vi "Exercise2.3-Data Acquisition - AM.vi"() -> ()   [LabVIEW 2013]
uses:
  <vilib>/Analysis/4window.llb/windowTd.ctl
  <vilib>/measure/maspectr.llb/FFT Power Spectrum and PSD for 1 Chan (CDB).vi
  <instrlib>/rtlsdr/rtlsdr.lvlib
  <vilib>/measure/NI_MAPro.lvlib
  <vilib>/Analysis/NI_AALPro.lvlib
panel:
  out "Spectrum":cluster{"f0":dbl, "df":dbl, "magnitude":dbl[]}(graph)={"f0"=104200000.0, "df"=24.414062499999996, "magnitude"=array[8192 elements]}
  out "XY Graph":cdb[](graph)
  in  "Samples Acquired":i32=16384
  out "error out":errorcluster
  in  "stop":bool
  out "error out":errorcluster
  out "DevRefnum":u64=294127816
  in  "center frequency":u32=104300000
  in  "sample rate":u32=200000
  # "FM 频谱扫描"
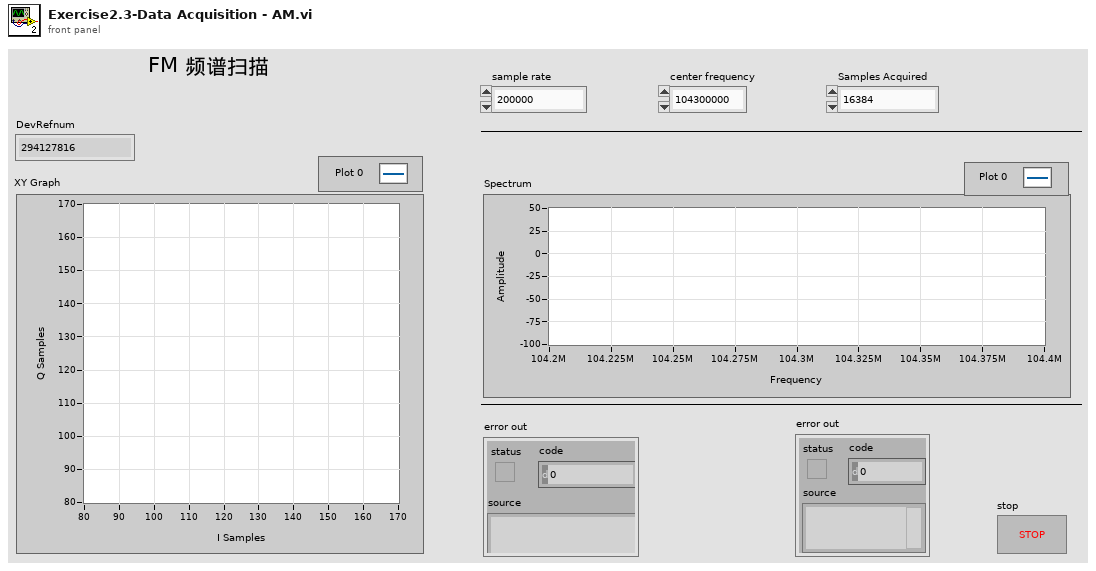
[diagram p1: front panel]
types:
  T1 = typedef "NI_AALPro.lvlib/windowTd.ctl" = u32
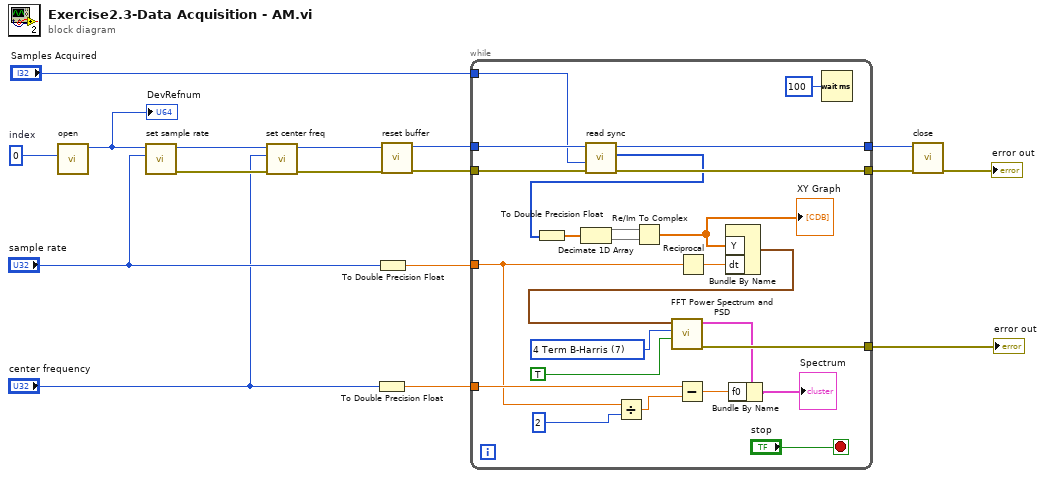
[diagram p0: block diagram]
diagram:
  w17 = u32 0  # index
  n1 = call <instrlib>:"open.vi"("index"=w17) -> ("DevRefnum"=w10:u64)  [unwired: 9 in, 1 out]
  "DevRefnum" <- w10
  n2 = call <instrlib>:"set sample rate.vi"("rate"="sample rate", "DevRefnum"=w10) -> ("error out"=w14:errorcluster, "DevRefnum"=w16:u64)  [unwired: 7 in, 1 out]
  n3 = call <instrlib>:"set center freq.vi"("error in (no error)"=w14, "freq"="center frequency", "DevRefnum"=w16) -> ("error out"=w13:errorcluster, "DevRefnum"=w15:u64)  [unwired: 6 in, 1 out]
  n4 = To Double Precision Float(number="center frequency") -> (double precision float=w2:dbl)
  n5 = To Double Precision Float(number="sample rate") -> (double precision float=w4:dbl)
  n6 = call <instrlib>:"reset buffer.vi"("error in (no error)"=w13, "DevRefnum"=w15) -> ("error out"=w11:errorcluster, "DevRefnum"=w9:u64)  [unwired: 8 in]
  n7 = while {
    tunnel: w11 -> [w41]
    tunnel: [w40] -> w12
    tunnel: w9 -> [w37]
    tunnel: [w36] -> w8
    tunnel: w2 -> [w29]
    tunnel: w4 -> [w27]
    tunnel: [w23] -> w6
    tunnel: "Samples Acquired" -> [w21]
    stop <- "stop" stop-if-true
    w35 = T1 7 items=["Rectangle"=0, "Hanning"=1, "Hamming"=2, "Blackman-Harris"=3, "Exact Blackman"=4, "Blackman"=5, "Flat Top"=6, "4 Term B-Harris "=7, "7 Term B-Harris"=8, "Low Sidelobe"=9, "Blackman Nuttall"=11, "Triangle"=30, "Bartlett-Hanning"=31, "Bohman"=32, "Parzen"=33, "Welch"=34, "Kaiser"=60, "Dolph-Chebyshev"=61, "Gaussian"=62] ("window")
    n8 = call <instrlib>:"read sync.vi"("error in (no error)"=w41, "len"=w21, "DevRefnum"=w37) -> ("error out"=w40:errorcluster, "buf 2"=w31:u8[], "DevRefnum"=w36:u64)  [unwired: 6 in]
    n9 = To Double Precision Float(number=w31) -> (double precision float=w39:dbl[])
    n10 = Decimate 1D Array "Decimate 1D Array"(w39) -> (w33:dbl[], w32:dbl[])
    n11 = Divide(x=w27, y=u32 2) -> (x/y=w25:dbl)
    n12 = Re/Im To Complex(1:w32, 2:w33) -> (0:w18:cdb[])
    "XY Graph" <- w18
    n13 = Subtract(x=w29, y=w25) -> (x-y=w30:dbl)
    n14 = Reciprocal(x=w27) -> (1/x=w28:dbl)
    n15 = Bundle By Name ("Build Waveform")("Y"=w18, "dt"=w28) -> (w20:waveform(cdb))  [unwired: 1 in]
    n16 = call-poly <vilib>:"FFT Power Spectrum and PSD.vi"("dB On (F)"=TRUE, "window"=w35, "time signal"=w20) -> ("error out"=w23:errorcluster, "Power Spectrum / PSD"=w22:cluster{"f0":dbl, "df":dbl, "magnitude":dbl[]})  [unwired: 5 in, 2 out]
    n17 = Bundle By Name(cluster=w22, "f0"=w30) -> (→"Spectrum":cluster{"f0":dbl, "df":dbl, "magnitude":dbl[]})
    n18 = Wait (ms)(milliseconds to wait=u32 100) -> ()  [unwired: 1 out]
  }
  "error out" <- w6
  n19 = call <instrlib>:"close.vi"("error in (no error)"=w12, "DevRefnum"=w8) -> ("error out"=→"error out":errorcluster)  [unwired: 8 in, 1 out]
